vi "Run.vi"(8 "error in (no error)":errorcluster, 9 "TestResult":refnum<class "TestResult.lvclass">, 10 "TestSuite":refnum<class "TestSuite.lvclass">, 11 "TestRunner in":refnum<class "TestRunner.lvclass">) -> (0 "error out":errorcluster, 1 "TestResult out":refnum<class "TestResult.lvclass">, 3 "TestRunner out":refnum<class "TestRunner.lvclass">)   [LabVIEW 2019, in "TestRunner.lvclass"]
uses:
  TestRunner.lvclass
  TestSuite/TestSuite.lvclass
  TestResult/TestResult.lvclass
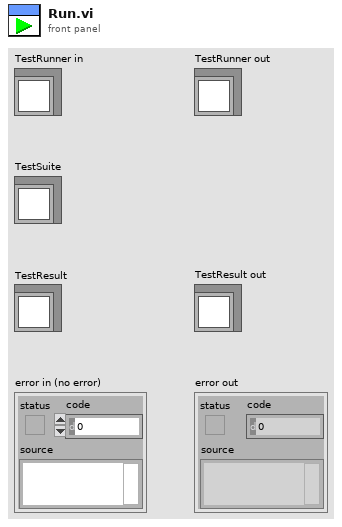
[diagram p1: front panel]
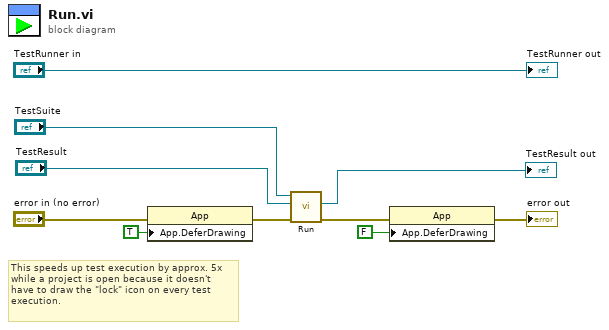
[diagram p0: block diagram]
diagram:
  # "This speeds up test execution by approx. 5x\nwhile a project is open because it doesn't\nhave to draw the \"lock\" icon on every test\nexecution."
  n1 = property class="App"(error in="error in (no error)", "App.DeferDrawing"=TRUE ("Application:Defer Drawing")) -> (error out=w6:errorcluster)  [unwired: 1 in, 1 out]
  n2 = call-dynamic "Run.vi"("error in (no error)"=w6, "TestResult"="TestResult", "TestSuite in"="TestSuite") -> ("error out"=w5:errorcluster, "TestResult out"=→"TestResult out":refnum<class "TestResult.lvclass">)  [unwired: 6 in, 1 out]
  n3 = property class="App"(error in=w5, "App.DeferDrawing"=FALSE ("Application:Defer Drawing")) -> (error out=→"error out":errorcluster)  [unwired: 1 in, 1 out]
  "TestRunner out" <- "TestRunner in"
